vi "RSZVB Get Port Impedances Renormalization.vi"(8 "error in (no error)":errorcluster {"code" format="%.0x"}, 10 "Channel (1)":i32=1, 11 "VISA session":refnum<visa-resource-name>) -> (0 "error out":errorcluster {"code" format="%.0x"}, 1 "Theory":i32, 3 "dup VISA session":refnum<visa-resource-name>)   [LabVIEW 2011]
doc: "This VI returns the theory for the renormalization of port impedances.\n\nRemote-control command(s):\nCALCulate<Chn>:TRANsform:IMPedance:RNORmal?"
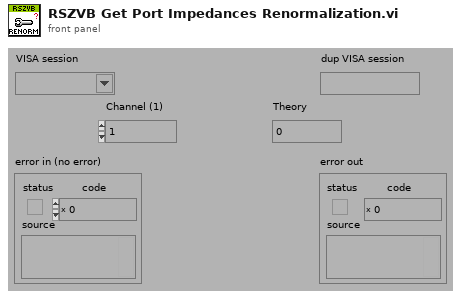
[diagram p1: front panel]
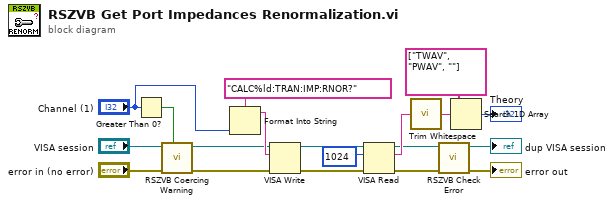
[diagram p0: block diagram]
diagram:
  n1 = Greater Than 0?(x="Channel (1)") -> (x > 0?=w17:bool)
  n2 = call "RSZVB Coercing Warning.vi"("In Range?"=w17, "error in (no error)"="error in (no error)", "VISA session"="VISA session") -> ("error out"=w16:errorcluster, "dup VISA session"=w18:refnum<visa-resource-name>)  [unwired: 7 in]
  n3 = Format Into String(format string="CALC%ld:TRAN:IMP:RNOR?", "Channel (1)") -> (resulting string=w19:string)  [unwired: 2 in, 1 out]
  n4 = VISA Write(VISA resource name=w18, write buffer=w19, error in (no error)=w16) -> (VISA resource name out=w10:refnum<visa-resource-name>, error out=w11:errorcluster)  [unwired: 1 out]
  n5 = VISA Read(VISA resource name=w10, byte count=u32 1024 ("byte count (0)"), error in (no error)=w11) -> (VISA resource name out=w4:refnum<visa-resource-name>, read buffer=w5:string, error out=w9:errorcluster)  [unwired: 1 out]
  n6 = call <vilib>:"Trim Whitespace.vi"("string"=w5) -> ("trimmed string"=w7:string)  [unwired: 1 in]
  n7 = call "RSZVB Check Error.vi"("error in (no error)"=w9, "VISA session"=w4) -> ("error out"=→"error out":errorcluster, "dup VISA session"=→"dup VISA session":refnum<visa-resource-name>)  [unwired: 8 in]
  n8 = Search 1D Array(1D array=string[] ["TWAV", "PWAV", ""], element=w7) -> (index of element=→"Theory":i32)  [unwired: 1 in]
